vi "Write pathname.vi"(8 "error in (no error)":errorcluster, 10 "pathname":string, 11 "Unix Pipe in":refnum<class "Unix Pipe.lvclass">) -> (0 "error out":errorcluster, 3 "Unix Pipe out":refnum<class "Unix Pipe.lvclass">)   [LabVIEW 2016, in "Linux RT IPC.Pipes.lvlib" / "Unix Pipe.lvclass"]
uses:
  Unix Pipe.lvclass
  Unix Pipe.lvclass/Unix Pipe.ctl
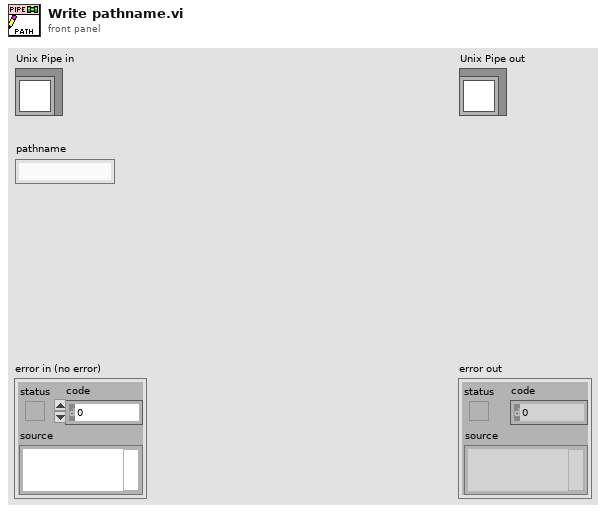
[diagram p1: front panel]
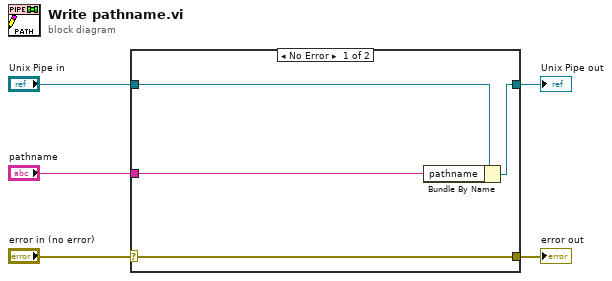
[diagram p0: block diagram]
diagram:
  n1 = case shown="No Error" "error in (no error)" {
    selector: "error in (no error)" -> [w9 w10]
    tunnel: [w9 w10] -> w4
    tunnel: [w7 w11] -> w2
    tunnel: "Unix Pipe in" -> [w8 w11]
    tunnel: "pathname" -> [w6 _]
    frame No Error {
      n2 = Bundle By Name(cluster=w8, "pathname"=w6) -> (w7:refnum<class "Unix Pipe.lvclass">)
    }
    frame Error {
    }
  }
  "error out" <- w4
  "Unix Pipe out" <- w2
